vi "Disconnect.vi"(8 "error in":errorcluster, 11 "MLTFNC in":refnum<class "MLTFNC.lvclass">) -> (0 "error out":errorcluster, 3 "MLTFNC out":refnum<class "MLTFNC.lvclass">)   [LabVIEW 2019, in "MLTFNC.lvlib" / "MLTFNC.lvclass"]
uses:
  Library/MLTFNC.lvclass
  builds/Instruments/Instruments.lvlibp/Library/Instruments.lvclass
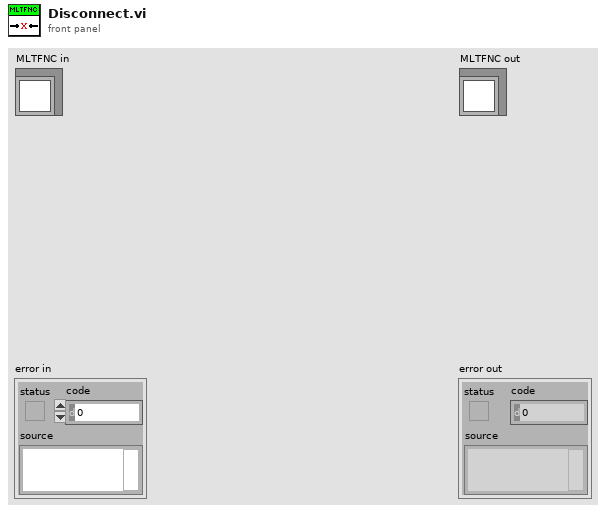
[diagram p1: front panel]
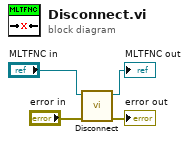
[diagram p0: block diagram]
diagram:
  n1 = call-parent "Disconnect.vi"("error in"="error in", "Instruments in"="MLTFNC in") -> ("error out"=→"error out":errorcluster, "Instruments out"=→"MLTFNC out":refnum<class "MLTFNC.lvclass">)  [unwired: 8 in]
